vi "normal display to hex display.vi"(6 "Normal display":string) -> (2 "Hex display":string)   [LabVIEW 2015]
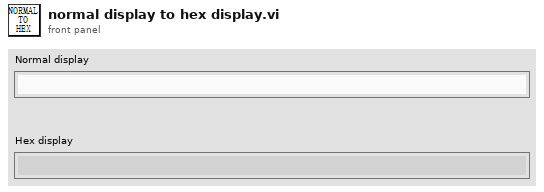
[diagram p1: front panel]
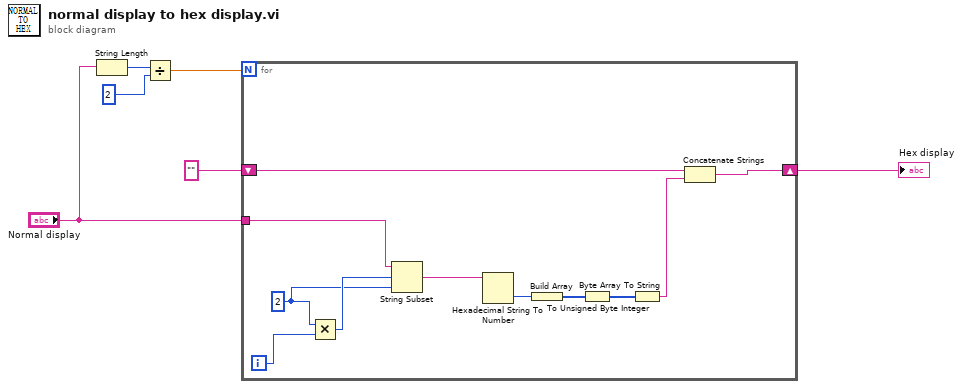
[diagram p0: block diagram]
diagram:
  n1 = String Length(string="Normal display") -> (length=w3:i32)
  n2 = Divide(x=w3, y=2) -> (x/y=w1:dbl)
  n3 = for {
    N: w1 -> [_]
    tunnel: "Normal display" -> [w14]
    shift-right: [w10] -> w5
    shift-left: "" -> [w11]
    i -> [w17]
    w15 = 2
    n4 = Multiply(x=w15, y=w17) -> (x*y=w16:i32)
    n5 = String Subset(string=w14, offset (0)=w16, length (rest)=w15) -> (substring=w13:string)
    n6 = Hexadecimal String To Number(string=w13) -> (number=w9:u32)  [unwired: 2 in, 1 out]
    n7 = Build Array(w9) -> (w8:u32[])
    n8 = To Unsigned Byte Integer(number=w8) -> (unsigned 8bit integer=w7:u8[])
    n9 = Byte Array To String(unsigned byte array=w7) -> (string=w12:string)
    n10 = Concatenate Strings(w11, w12) -> (w10:string)
  }
  "Hex display" <- w5
